vi "combo_box_input.vi"(7 "callee":refnum<vi>, 8 "error in (no error)":errorcluster, 11 "configuration":T1) -> (0 "error out":errorcluster, 2 "value":string, 3 "dialog_selection":T2)   [LabVIEW 2015, in "lv-dialog-interfaces.lvlib"]
uses:
  lv-dialog-interfaces.lvlib
  <userlib>/antonio-alexander/lv-dialog/api/v1/public/_controls/selection.ctl
  private/_controls/dialog_type.ctl
  private/_controls/hmi_references.ctl
  private/_controls/configuration.ctl
  <vilib>/event_ctls.llb/eventvkey.ctl
  <userlib>/antonio-alexander/lv-dialog/api/v1/v1.lvlib
panel:
  out "dialog":string
  in  "combo_box":string(combo)
  in  "button_1":bool
  in  "button_2":bool
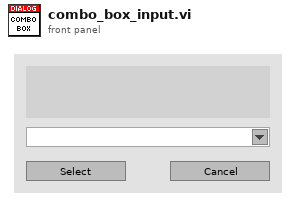
[diagram p1: front panel]
types:
  T1 = cluster{"dialog_text":string, "boolean_text_1":string, "boolean_text_2":string, "combo_box []":string[], "custom_entry":bool}
  T2 = typedef "lv-dialog.lvlib/v1.lvlib/selection.ctl" = enum16{"null", "panel_closed", "button_1", "button_2", "button_3", "cancelled"}
  T3 = typedef "lv-dialog-interfaces.lvlib/dialog_type.ctl" = enum16{"null", "one_button", "two_button", "three_button", "confirmation", "busy_wait", "error", "busy_wait_embed", "combo_box", "data_entry_string", "data_entry_numeric"}
  T4 = typedef "lv-dialog-interfaces.lvlib/configuration.ctl" = cluster{"dialog_text":string, "boolean_text_1":string, "boolean_text_2":string, "boolean_text_3":string, "inner_color":u32, "outer_color":u32, "wait_s":dbl, "error_status":bool, "error_source":string, "error_details":string, "string []":string[], "custom_entry":bool}
  T5 = typedef "lv-dialog-interfaces.lvlib/hmi_references.ctl" = cluster{"vi_reference":refnum<vi>, "caller":refnum<vi>, "dialog":refnum<vi>, "button_1":refnum<vi>, "button_2":refnum<vi>, "button_3":refnum<vi>, "busy":refnum<vi>, "error_glyph":refnum<vi>, "error_source":refnum<vi>, "error_text":refnum<vi>, "combo_box":refnum<vi>}
  T6 = typedef "eventvkey.ctl" = enum16{"ASCII", "Enter", "Return", "Shift", "Ctrl", "Alt", "Cmd", "Opt", "Caps", "NumLock", "Clear", "Break", "Up", "Down", "Left", "Right", "Insert", "Delete", "Home", "End", "PageUp", "PageDown", "Escape", "Help", "Pause", "ScrollLock", "F1", "F2", "F3", "F4", "F5", "F6", "F7", "F8", "F9", "F10", "F11", "F12", "F13", "F14", "F15", "F16", "F17", "F18", "F19", "F20", "F21", "F22", "F23", "F24", "Play", "VolumeUp", "VolumeDown", "Mute", "Two Byte Char"}
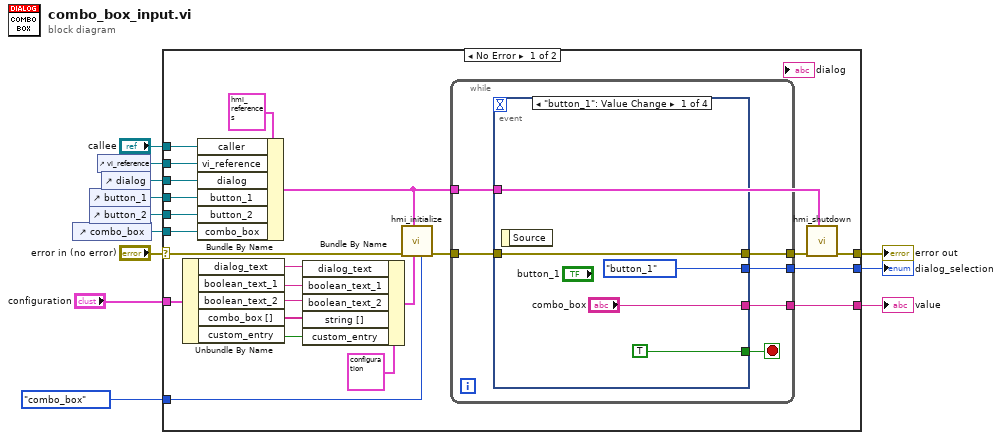
[diagram p0: block diagram]
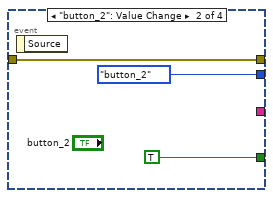
[diagram p2: hidden frame]
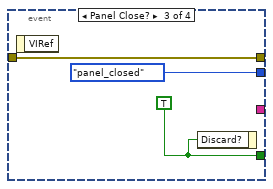
[diagram p3: hidden frame]
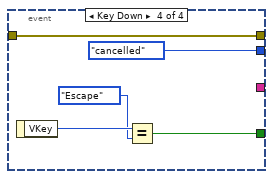
[diagram p4: hidden frame]
diagram:
  n1 = control-ref of="combo_box"() -> (w3:refnum<vi>)
  n2 = control-ref of="button_1"() -> (w5:refnum<vi>)
  n3 = control-ref of="button_2"() -> (w4:refnum<vi>)
  n4 = control-ref of="vi_reference"() -> (w7:refnum<vi>)
  n5 = control-ref of="dialog"() -> (w6:refnum<vi>)
  n6 = case shown="No Error" "error in (no error)" {
    selector: "error in (no error)" -> [w35 w57]
    tunnel: dialog_type."combo_box" ("dialog_type") -> [w34 _]
    tunnel: [w32 _] -> w10
    tunnel: "callee" -> [w31 _]
    tunnel: [w29 w57] -> w8
    tunnel: w7 -> [w28 _]
    tunnel: w6 -> [w23 _]
    tunnel: w5 -> [w24 _]
    tunnel: w4 -> [w25 _]
    tunnel: w3 -> [w26 _]
    tunnel: [w22 _] -> w2
    tunnel: "configuration" -> [w19 _]
    frame No Error {
      n7 = Unbundle By Name(w19) -> ("dialog_text"=w17:string, "boolean_text_1"=w16:string, "boolean_text_2"=w15:string, "combo_box []"=w18:string[], "custom_entry"=w13:bool)
      n8 = Bundle By Name(cluster=T5 {"vi_reference"=refnum, "caller"=refnum, "dialog"=refnum, "button_1"=refnum, "button_2"=refnum, "button_3"=refnum, "busy"=refnum, "error_glyph"=refnum, "error_source"=refnum, "error_text"=refnum, "combo_box"=refnum}, "caller"=w31, "vi_reference"=w28, "dialog"=w23, "button_1"=w24, "button_2"=w25, "combo_box"=w26) -> (w14:T5)
      n9 = Bundle By Name(cluster=T4 {"dialog_text"="", "boolean_text_1"="", "boolean_text_2"="", "boolean_text_3"="", "inner_color"=16711680, "outer_color"=6618880, "wait_s"=nan, "error_status"=FALSE, "error_source"="", "error_details"="", "string []"=[], "custom_entry"=FALSE} ("configuration"), "dialog_text"=w17, "boolean_text_1"=w16, "boolean_text_2"=w15, "string []"=w18, "custom_entry"=w13) -> (w20:T4)
      n10 = call "hmi_initialize.vi"("dialog_type"=w34, "configuration"=w20, "references"=w14, "error in (no error)"=w35) -> ("error out"=w33:errorcluster)  [unwired: 7 in]
      n11 = while {
        tunnel: [w39] -> w32
        tunnel: w33 -> [w41]
        tunnel: [w40] -> w30
        tunnel: [w37] -> w22
        tunnel: w14 -> [w36]
        stop <- w38 stop-if-true
        n12 = event shown="[0] \"button_1\": Value Change" {
          selector: _ -> [_ _ _ _]
          dyn-events: _ -> [_ _ _ _]
          timeout: _ -> [_ _ _ _]
          tunnel: w41 -> [w45 w48 w51 w56]
          tunnel: [w45 w48 w51 w56] -> w40
          tunnel: [selection."button_1" ("dialog_selection") selection."button_2" ("dialog_selection") selection."panel_closed" ("dialog_selection") selection."cancelled" ("dialog_selection")] -> w39
          tunnel: w36 -> [_ _ _ _]
          tunnel: [TRUE ("Discard?") TRUE ("Discard?") w49 w54] -> w38
          tunnel: ["combo_box" _ _ _] -> w37
          event "button_1": Value Change {
            n13 = event-data() -> ()  [unwired: 1 in, 1 out]
          }
          event "button_2": Value Change {
            n14 = event-data() -> ()  [unwired: 1 in, 1 out]
          }
          event Panel Close? {
            w49 = TRUE ("Discard?")
            n15 = event-data() -> ()  [unwired: 1 in, 1 out]
            n16 = event-data("Discard?"=w49) -> ()  [unwired: 1 in, 1 out]
          }
          event Key Down {
            n17 = event-data() -> ("VKey"=w53:T6)  [unwired: 1 in]
            n18 = Equal?(x=w53, y=eventvkey."Escape" ("VKey")) -> (x = y?=w54:bool)
          }
        }
      }
      n19 = call "hmi_shutdown.vi"("references"=w14, "error in (no error)"=w30) -> ("error out"=w29:errorcluster)  [unwired: 9 in]
    }
    frame Error {
    }
  }
  "error out" <- w8
  "dialog_selection" <- w10
  "value" <- w2
